vi "post_dust_source_small.vi"(8 "error in (no error)":errorcluster, 11 "Dust control settings":T1={"Integer Timestamp"=8, "Needle Voltage"=2.0, "Frequency"=3.0, "Width (ms) : 0.1 "=4.0, "Desired Amplitude (V)"=5.0, "Settings ID"="", "ID#"=7} {"Needle Voltage" min=0.0 max=10.0 step=0.01 format="%.2g"; "Desired Amplitude (V)" min=0.0 max=10.0 step=0.01 format="%5.2f"; "Width (ms) : 0.1" min=0.05 max=5.0 step=0.01 format="%6.2f"; "Frequency" min=1.0 max=100.0 step=0.01 format="%.1f"}) -> (0 "error out":errorcluster)   [LabVIEW 2013]
doc: "Adds a new row to the source_settings table."
uses:
  Small Accelerator/dust_source_control_small.ctl
  <vilib>/addons/database/NI_Database_API.lvlib
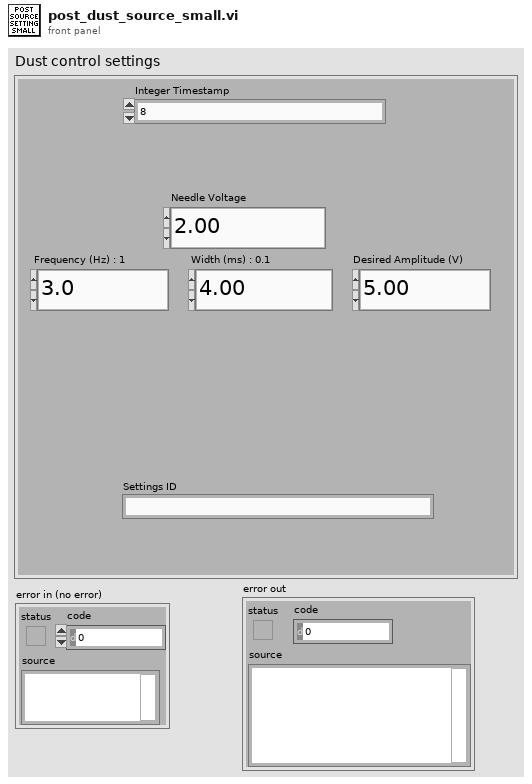
[diagram p1: front panel]
types:
  T1 = typedef "dust_source_control_small.ctl" = cluster{"Integer Timestamp":u64, "Needle Voltage":dbl, "Frequency":dbl, "Width (ms) : 0.1 ":dbl, "Desired Amplitude (V)":dbl, "Settings ID":string, "ID#":i32}
  T2 = typedef "NI_Database_API.lvlib/Conn ObjectReference.ctl" = refnum<k1>
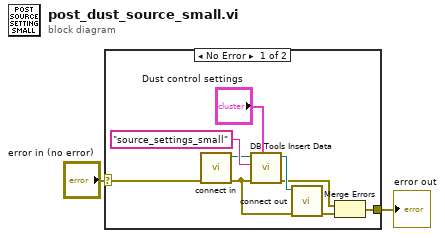
[diagram p0: block diagram]
diagram:
  n1 = case shown="No Error" "error in (no error)" {
    selector: "error in (no error)" -> [w11 w12]
    tunnel: [w3 w12] -> w1
    frame No Error {
      n2 = call "connect in.vi"("error in (no error)"=w11) -> ("error out"=w5:errorcluster, "Database Connection"=w9:T2)  [unwired: 6 in, 1 out]
      n3 = call <vilib>:"DB Tools Insert Data.vi"("data"="Dust control settings", "error in (no error)"=w5, "table"="source_settings_small", "connection reference"=w9) -> ("error out"=w6:errorcluster, "connection reference out"=w8:T2)  [unwired: 6 in]
      n4 = call "connect out.vi"("error in (no error)"=w5, "connection reference"=w8) -> ("error out"=w4:errorcluster)  [unwired: 9 in]
      n5 = Merge Errors(w6, w4) -> (w3:errorcluster)
    }
    frame Error {
    }
  }
  "error out" <- w1
